vi "temperature.vi"() -> ()   [LabVIEW 2022 SP3]
panel:
  out "Waveform Graph":dbl[](graph)
  out "Waveform Chart":dbl(graph)
  in  "stop":bool
  in  "Slide":dbl(slide) scale=0.0..200.0
  out "Thermometer":dbl(slide) scale=0.0..600.0
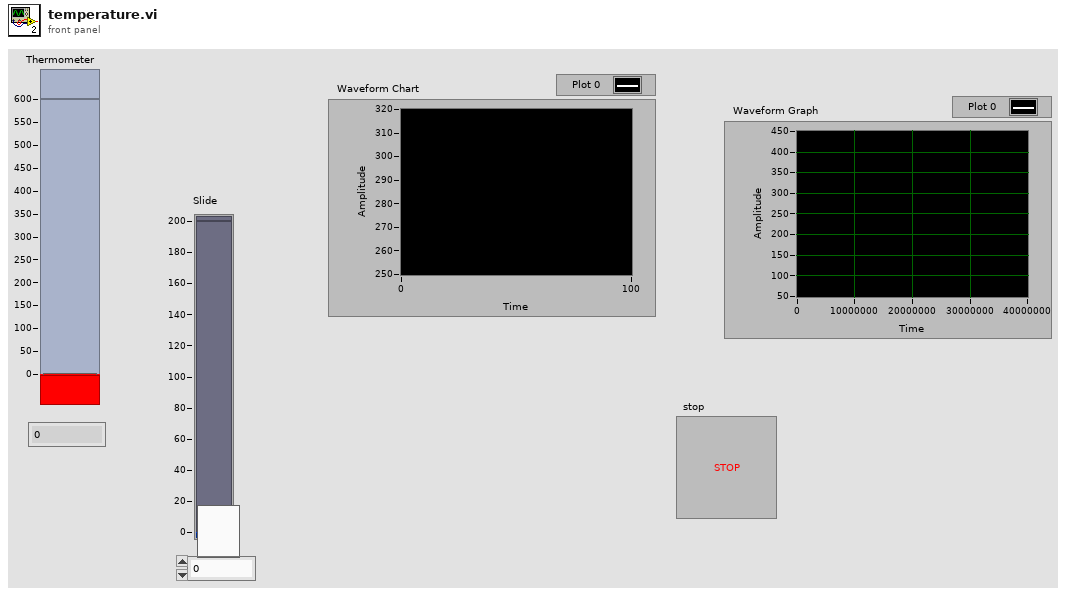
[diagram p1: front panel]
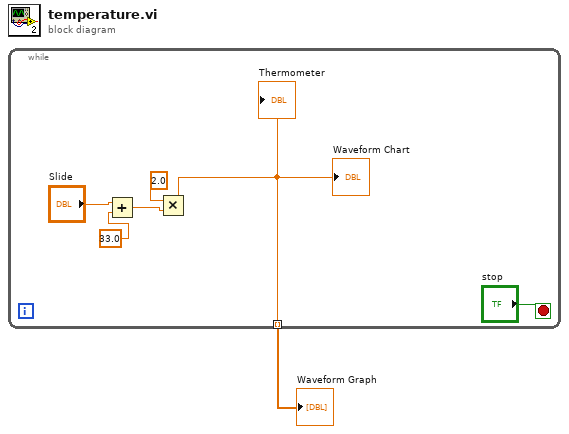
[diagram p0: block diagram]
diagram:
  n1 = while {
    tunnel: [w2] -> w1 mode=indexing
    stop <- "stop" stop-if-true
    n2 = Add(x="Slide", y=33.0) -> (x+y=w5:dbl)
    n3 = Multiply(x=2.0, y=w5) -> (x*y=w2:dbl)
    "Thermometer" <- w2
    "Waveform Chart" <- w2
  }
  "Waveform Graph" <- w1
